vi "Display_Values.vi"(8 "error in (no error)":errorcluster, 9 "Data in":T1 {"Shaft"."dmin" format="%#_7g"; "Shaft"."dmax" format="%#_7g"; "Shaft"."Fundamental Dev" format="%#_7g"; "Shaft"."Tolerance Grade (IT) Shaft" format="%#_7g"; "Hole"."Dmin" format="%#_7g"; "Hole"."Tolerance Grade (IT)" format="%#_7g"}, 10 "Shaft":refnum<vi>, 11 "Hole":refnum<vi>) -> (0 "error out":errorcluster, 3 "Data out":T1 {"Shaft"."dmin" format="%#_7g"; "Shaft"."dmax" format="%#_7g"; "Shaft"."Fundamental Dev" format="%#_7g"; "Shaft"."Tolerance Grade (IT) Shaft" format="%#_7g"; "Hole"."Dmin" format="%#_7g"; "Hole"."Tolerance Grade (IT)" format="%#_7g"})   [LabVIEW 2023]
uses:
  TypeDef/Data_Cluster.ctl
  TypeDef/Units.ctl
  TypeDef/Method_Info.ctl
  TypeDef/Hole_Data.ctl
  TypeDef/Shaft_Data.ctl
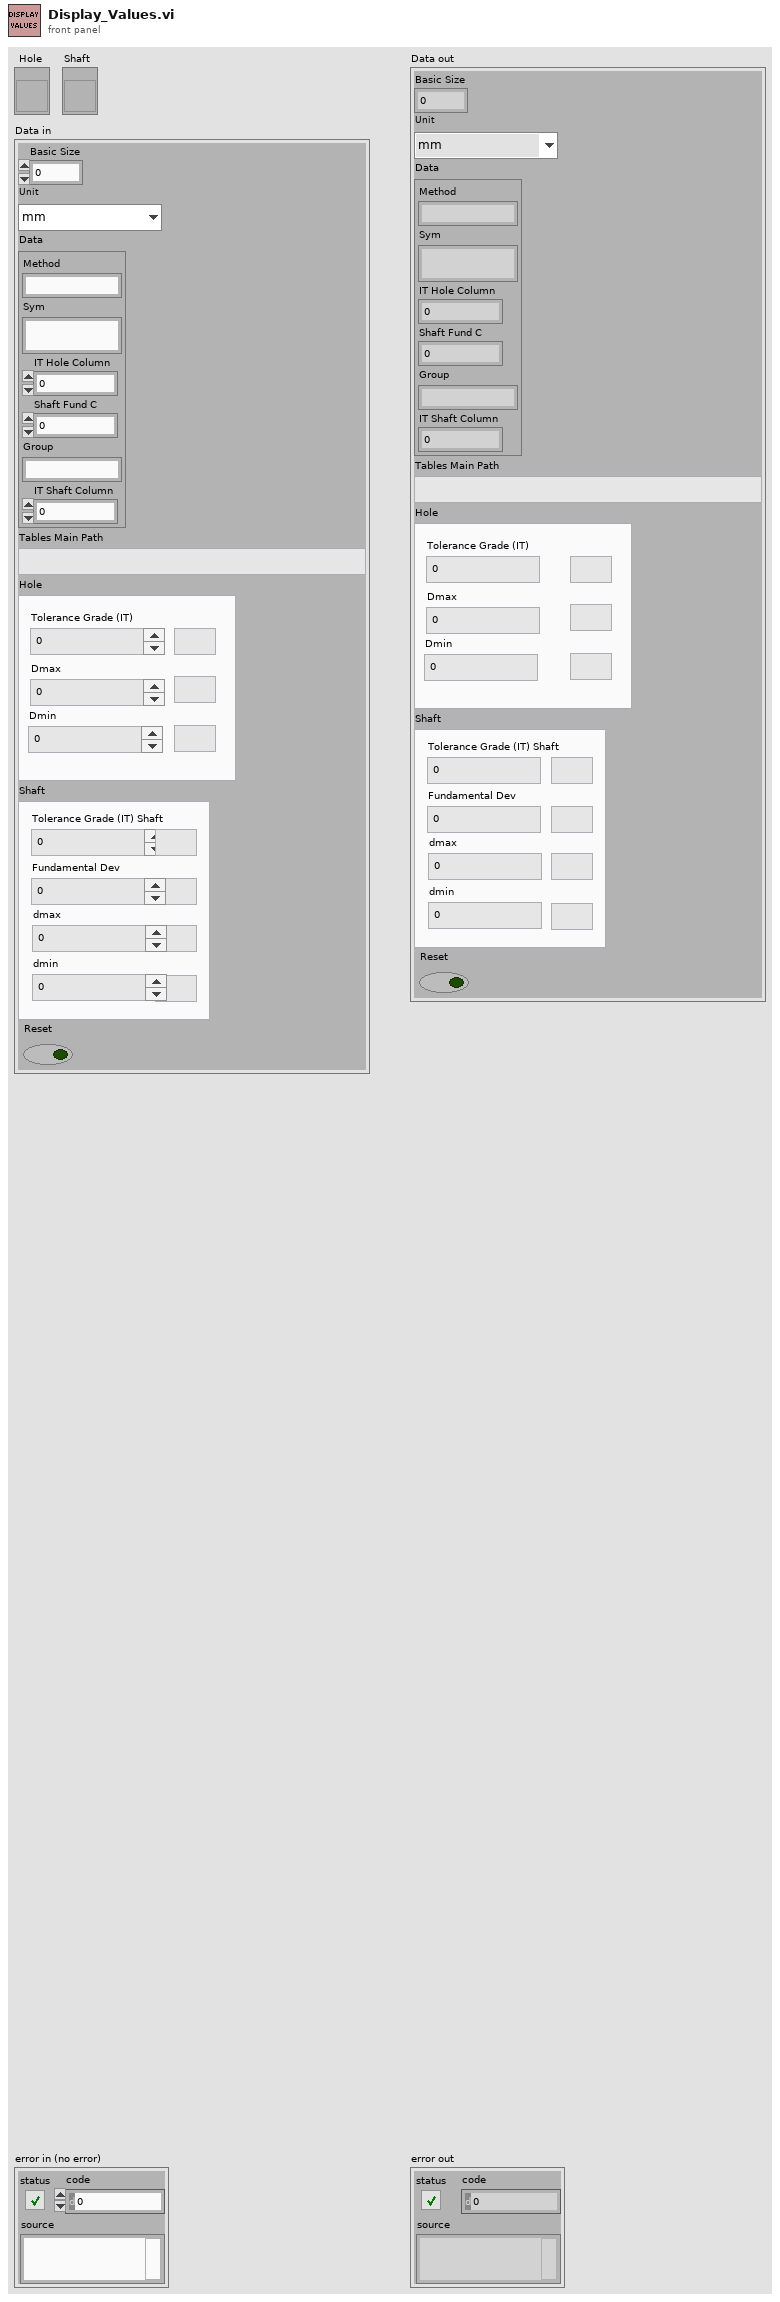
[diagram p1: front panel]
types:
  T1 = typedef "Data_Cluster.ctl" = cluster{"Basic Size ":dbl, "Unit":T2, "Data":T3, "Tables Main Path":path, "Hole":T4, "Shaft":T5, "Reset":bool}
  T2 = typedef "Units.ctl" = enum16{"mm", "in"}
  T3 = typedef "Method_Info.ctl" = cluster{"Method":string, "Sym":string, "IT Hole Column":i32, "Shaft Fund C":i32, "Group":string, "IT Shaft Column":i32}
  T4 = typedef "Hole_Data.ctl" = cluster{"Tolerance Grade (IT)":dbl, "Dmax":dbl, "Units Hole":cluster{"units_it":string, "units_Dmax\nUnits_Dmax":string, "Units_Dmin":string}, "Dmin":dbl}
  T5 = typedef "Shaft_Data.ctl" = cluster{"Tolerance Grade (IT) Shaft":dbl, "Units Shaft":cluster{"Units_FundamentalDev":string, "Units_dmax":string, "Units_dmin":string, "Units_IT_Shaft":string}, "Fundamental Dev":dbl, "dmax":dbl, "dmin":dbl}
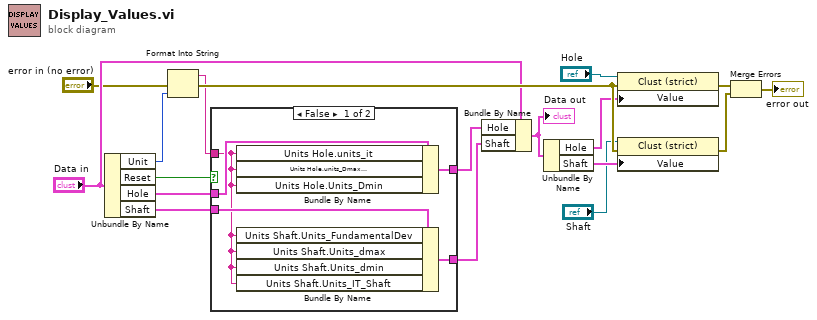
[diagram p0: block diagram]
diagram:
  n1 = Unbundle By Name("Data in") -> ("Unit"=w7:T2, "Reset"=w6:bool, "Hole"=w3:T4, "Shaft"=w2:T5)
  n2 = Format Into String(error in="error in (no error)", w7) -> (resulting string=w10:string, error out=w16:errorcluster)  [unwired: 2 in]
  n3 = case shown="False" w6 {
    tunnel: w10 -> [w19 _]
    tunnel: [w21 _] -> w4
    tunnel: w3 -> [w23 _]
    tunnel: w2 -> [w22 _]
    tunnel: [w20 _] -> w1
    frame False {
      n4 = Bundle By Name(cluster=w23, "Units Hole.units_it"=w19, "Units Hole.units_Dmax\nUnits_Dmax"=w19, "Units Hole.Units_Dmin"=w19) -> (w21:T4)
      n5 = Bundle By Name(cluster=w22, "Units Shaft.Units_FundamentalDev"=w19, "Units Shaft.Units_dmax"=w19, "Units Shaft.Units_dmin"=w19, "Units Shaft.Units_IT_Shaft"=w19) -> (w20:T5)
    }
    frame True {
    }
  }
  n6 = Bundle By Name(cluster="Data in", "Hole"=w4, "Shaft"=w1) -> (w5:T1)
  "Data out" <- w5
  n7 = Unbundle By Name(w5) -> ("Hole"=w13:T4, "Shaft"=w15:T5)
  n8 = property class="Clust (strict)"(reference="Hole", error in=w16, "Value"=w13) -> (error out=w12:errorcluster)  [unwired: 1 out]
  n9 = property class="Clust (strict)"(reference="Shaft", error in=w16, "Value"=w15) -> (error out=w18:errorcluster)  [unwired: 1 out]
  n10 = Merge Errors(w12, w18) -> (→"error out":errorcluster)
